vi "GetPythonFunction.vi"(5 "function name":string, 6 "error in":errorcluster, 9 "PythonConverter in":refnum<class "PythonBDConverter.lvclass">) -> (0 "error out":errorcluster, 3 "PythonConverter out":refnum<class "PythonBDConverter.lvclass">, 4 "Python function":refnum<class "PythonFunction.lvclass">)   [LabVIEW 2014, in "PythonBDConverter.lvclass"]
uses:
  PythonBDConverter.lvclass
  Parsing/Classes/PythonFunction/PythonFunction.lvclass
  PythonBDConverter.lvclass/PythonBDConverter.ctl
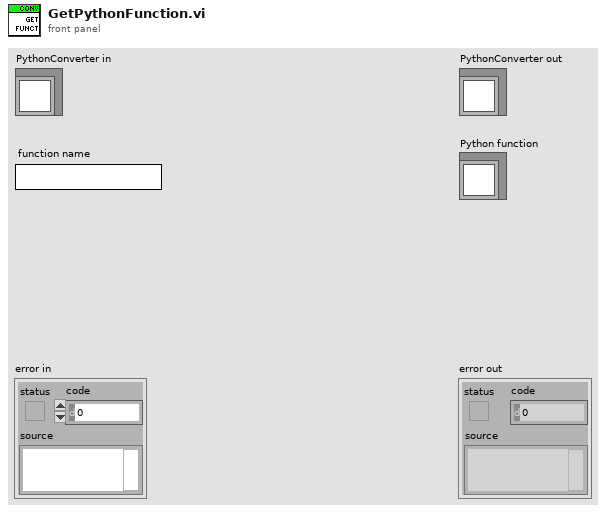
[diagram p1: front panel]
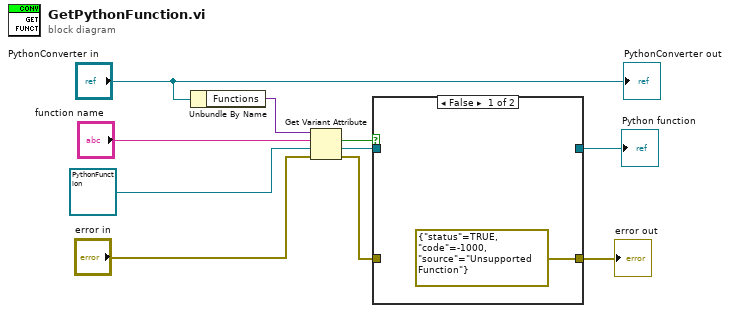
[diagram p0: block diagram]
diagram:
  n1 = Unbundle By Name("PythonConverter in") -> ("Functions"=w10:variant)
  n2 = Get Variant Attribute(Variant=w10, name="function name", default value (empty Variant)=refnum<class "PythonFunction.lvclass"> refnum ("Python function"), error in="error in") -> (found=w6:bool, value=w2:refnum<class "PythonFunction.lvclass">, error out=w4:errorcluster)  [unwired: 1 out]
  n3 = case shown="False" w6 {
    tunnel: w4 -> [_ w13]
    tunnel: [errorcluster {"status"=TRUE, "code"=-1000, "source"="Unsupported Function"} ("error out") w13] -> w3
    tunnel: w2 -> [_ w12]
    tunnel: [_ w12] -> w1
    frame False {
    }
    frame True {
    }
  }
  "error out" <- w3
  "Python function" <- w1
  "PythonConverter out" <- "PythonConverter in"
